vi "From Single.vi"(4 "CmdDigital":T2) -> (7 "CmdDigitalMultiple":T1)   [LabVIEW 2023, in "CmdDigitalMultiple.lvlib"]
uses:
  CmdDigitalMultiple.lvlib
  CmdDigital/Data.ctl
  CmdDigital/CmdDigital.lvlib
  Data.ctl
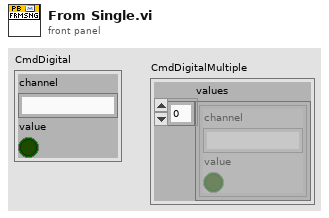
[diagram p1: front panel]
types:
  T1 = typedef "CmdDigitalMultiple.lvlib/Data.ctl" = cluster{"values":T2[]}
  T2 = typedef "CmdDigital.lvlib/Data.ctl" = cluster{"channel":string, "value":bool}
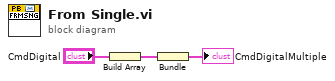
[diagram p0: block diagram]
diagram:
  n1 = Build Array("CmdDigital") -> (w2:T2[])
  n2 = Bundle(w2) -> (→"CmdDigitalMultiple":cluster{T2[]})  [unwired: 1 in]
